vi "Data Type to I32 1D.vi"(8 "error in (no error)":errorcluster, 11 "Data Type":refnum<class "Data Type.lvclass">) -> (0 "error out":errorcluster, 3 "I32 1D out":i32[](array[numeric]))   [LabVIEW 2019, in "I32 1D.lvclass"]
uses:
  <vilib>/gpm_packages/@cs/data-type-serializer/source/I32 1D/I32 1D.lvclass
  <vilib>/gpm_packages/@cs/data-type-serializer/source/Data Type/Data Type.lvclass
  <vilib>/gpm_packages/@cs/data-type-serializer/source/I32 1D/I32 1D.lvclass/I32 1D.ctl
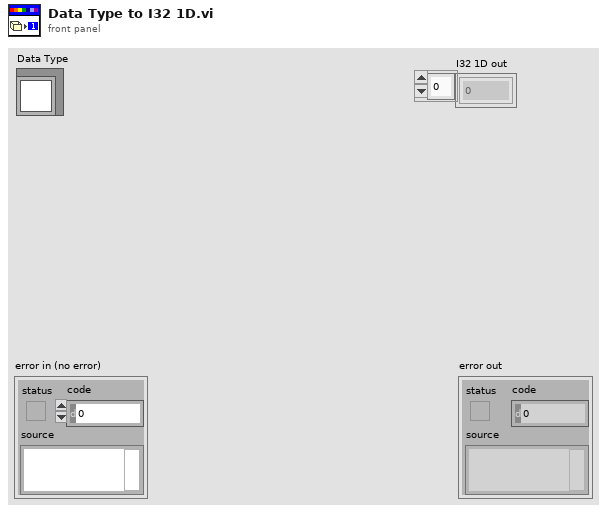
[diagram p1: front panel]
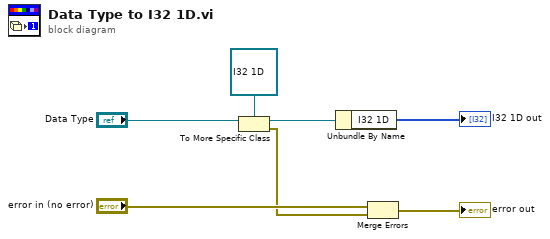
[diagram p0: block diagram]
diagram:
  n1 = To More Specific Class(target class=refnum<class "I32 1D.lvclass"> refnum ("Boolean out"), reference="Data Type") -> (specific class reference=w4:refnum<class "I32 1D.lvclass">, error out=w2:errorcluster)  [unwired: 1 in]
  n2 = Unbundle By Name(w4) -> ("I32 1D"=→"I32 1D out":i32[])
  n3 = Merge Errors("error in (no error)", w2) -> (→"error out":errorcluster)
